vi "Exit.vi"(8 "error in (no error)":errorcluster, 10 "Context in":refnum<class "Context.lvclass">, 11 "Active in":refnum<class "Active.lvclass">) -> (0 "error out":errorcluster, 2 "Context out":refnum<class "Context.lvclass">, 3 "Active out":refnum<class "Active.lvclass">)   [LabVIEW 2024, in "State.lvlib" / "Active.lvclass"]
uses:
  Active.lvclass
  Context/Context/Context.lvclass
  Active.lvclass/Active.ctl
panel:
  # "EXIT ACTIVE"
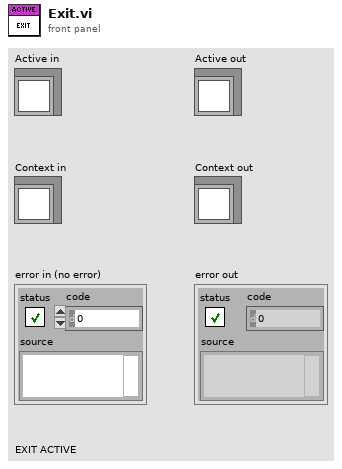
[diagram p1: front panel]
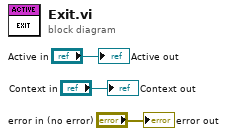
[diagram p0: block diagram]
diagram:
  "error out" <- "error in (no error)"
  "Active out" <- "Active in"
  "Context out" <- "Context in"
